vi "EXA_logEvent_HeartbeatIn.vi"(8 "error in (no error)":errorcluster, 11 "logevent_HeartbeatIn_Ctl":T1) -> (0 "error out":errorcluster, 2 "function return":i32, 3 "logevent_HeartbeatIn_Ctl out":T1)   [LabVIEW 2016, in "SALLV_EXA.lvlib"]
doc: "int EXA_shm_logEvent_HeartbeatInLV(EXA_logevent_HeartbeatInLV *logevent_HeartbeatIn_Ctl );"
uses:
  SALLV_EXA.lvlib
  DataTypes/logevent_HeartbeatIn.ctl
  SALLV_EXA.so
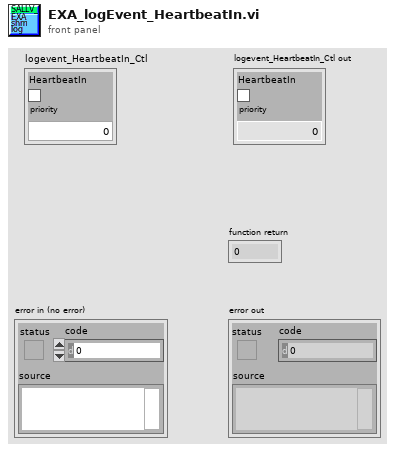
[diagram p1: front panel]
types:
  T1 = typedef "SALLV_EXA.lvlib/logevent_HeartbeatIn.ctl" = cluster{"HeartbeatIn":bool, "priority":i32}
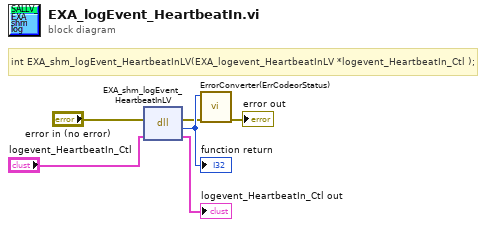
[diagram p0: block diagram]
diagram:
  # "int EXA_shm_logEvent_HeartbeatInLV(EXA_logevent_HeartbeatInLV *logevent_HeartbeatIn_Ctl );"
  n1 = dll-call lib="home/andres/Desktop/ts_sallv_EXA2/SALLV_EXA.*" fn="EXA_shm_logEvent_HeartbeatInLV"(error in="error in (no error)", "logevent_HeartbeatIn_Ctl"="logevent_HeartbeatIn_Ctl") -> (error out=w2:errorcluster, w6:i32, "logevent_HeartbeatIn_Ctl"=→"logevent_HeartbeatIn_Ctl out":T1)  [unwired: 2 in, 1 out]
  "function return" <- w6
  n2 = call "ErrorConverter(ErrCodeorStatus).vi"("error in (no error)"=w2, "error code"=w6) -> ("error out"=→"error out":errorcluster)  [unwired: 9 in]
